vi "CalibrateCurrentDriver.vi"() -> ()   [LabVIEW 2025]
uses:
  <vilib>/Analysis/1siggen.llb/Ramp Pattern by Samples.vi
  <vilib>/Analysis/NI_AALBase.lvlib
  instr.lib/Keithley 648X Series/Keithley 648X Series.lvlib
  <userlib>/_OpenG.lib/time/time.llb/openg_time.lvlib
  <vilib>/Analysis/NI_AALPro.lvlib
panel:
  out "Resistance":dbl format="%#_6p"
  out "intercept":dbl format="%^#_6g"
  out "slope":dbl format="%^#_6g"
  out "XY Graph":cluster{dbl[], "Ramp Pattern":dbl[]}(graph)
  in  "milliseconds to wait":u32
  in  "VISA resource name":refnum<visa-resource-name>
  in  "VSource":refnum<k21>
  in  "nSteps":i32=100 min=2 max=1000 step=1
  in  "MaxVolts":dbl=10.0
  in  "MinVolts":dbl
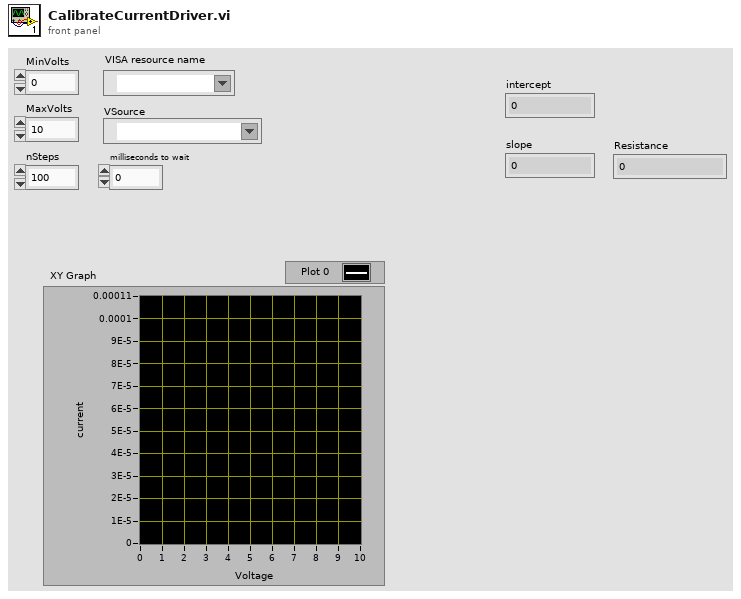
[diagram p1: front panel]
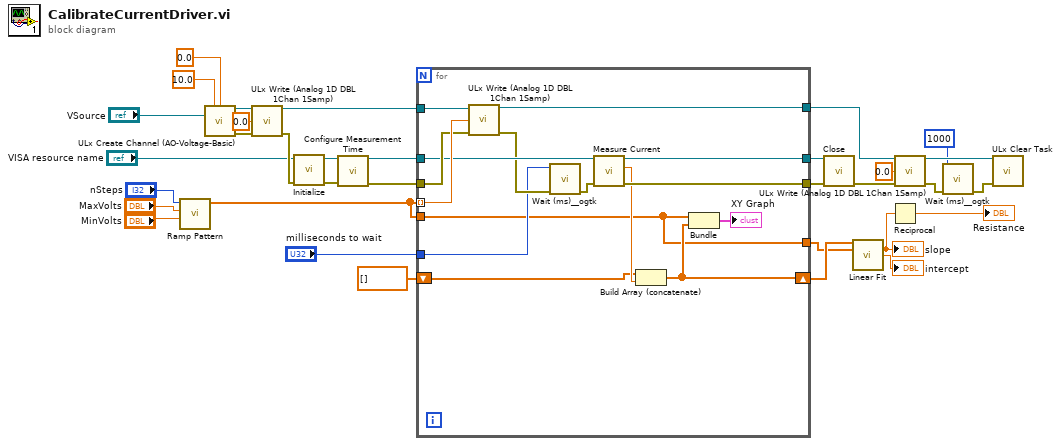
[diagram p0: block diagram]
diagram:
  n1 = call-poly <vilib>:"Ramp Pattern.vi"("start"="MinVolts", "end"="MaxVolts", "samples"="nSteps") -> ("Ramp Pattern"=w13:dbl[])  [unwired: 7 in, 1 out]
  n2 = call <instrlib>:"ULx Create Channel (AO-Voltage-Basic).vi"("maximum value"=10.0, "minimum value"=0.0, "physical channels"="VSource") -> ("task out"=w27:refnum<k24>, "error out"=w26:errorcluster)  [unwired: 11 in]
  n3 = call <instrlib>:"ULx Write (Analog 1D DBL 1Chan 1Samp).vi"("task in"=w27, "data"=0.0, "error in"=w26) -> ("task out"=w18:refnum<k24>, "error out"=w24:errorcluster)  [unwired: 10 in, 1 out]
  n4 = call "Initialize.vi"("error in (no error)"=w24, "VISA resource name"="VISA resource name") -> ("error out"=w21:errorcluster, "VISA resource name out"=w22:refnum<visa-resource-name>)  [unwired: 8 in]
  n5 = call "Configure Measurement Time.vi"("VISA resource name"=w22, "error in (no error)"=w21) -> ("VISA resource name out"=w19:refnum<visa-resource-name>, "error out"=w20:errorcluster)  [unwired: 12 in]
  n6 = for {
    tunnel: w20 -> [w46]
    tunnel: w19 -> [w45]
    tunnel: w18 -> [w48]
    tunnel: w13 -> [w47] mode=indexing
    tunnel: [w43] -> w16
    tunnel: "milliseconds to wait" -> [w41]
    tunnel: [w40] -> w15
    tunnel: [w39] -> w5
    shift-right: [w35] -> w12
    shift-left: dbl[] [] -> [w37]
    tunnel: w13 -> [w34]
    tunnel: [w34] -> w11
    n7 = call <instrlib>:"ULx Write (Analog 1D DBL 1Chan 1Samp).vi"("task in"=w48, "data"=w47, "error in"=w46) -> ("task out"=w39:refnum<k24>, "error out"=w44:errorcluster)  [unwired: 10 in, 1 out]
    n8 = call <userlib>:"Wait (ms)__ogtk.vi"("error in (no error)"=w44, "milliseconds to wait"=w41) -> ("error out"=w42:errorcluster)  [unwired: 8 in, 1 out]
    n9 = call "Measure Current.vi"("VISA resource name"=w45, "error in (no error)"=w42) -> ("VISA resource name out"=w43:refnum<visa-resource-name>, "Measurement"=w38:dbl, "error out"=w40:errorcluster)  [unwired: 11 in]
    n10 = Build Array (concatenate)(w37, w38) -> (w35:dbl[])
    n11 = Bundle("Ramp Pattern"=w34, w35) -> (→"XY Graph":cluster{"Ramp Pattern":dbl[], dbl[]})  [unwired: 1 in]
  }
  n12 = call "Close.vi"("error in (no error)"=w15, "VISA resource name"=w16) -> ("error out"=w4:errorcluster)  [unwired: 9 in]
  n13 = call <vilib>:"Linear Fit.vi"("Y"=w12, "X"=w11) -> ("slope"=w9:dbl, "intercept"=→"intercept":dbl)  [unwired: 9 in, 3 out]
  "slope" <- w9
  n14 = Reciprocal(x=w9) -> (1/x=→"Resistance":dbl)
  n15 = call <instrlib>:"ULx Write (Analog 1D DBL 1Chan 1Samp).vi"("task in"=w5, "data"=0.0, "error in"=w4) -> ("task out"=w6:refnum<k24>, "error out"=w3:errorcluster)  [unwired: 10 in, 1 out]
  n16 = call <userlib>:"Wait (ms)__ogtk.vi"("error in (no error)"=w3, "milliseconds to wait"=u32 1000) -> ("error out"=w2:errorcluster)  [unwired: 8 in, 1 out]
  n17 = call <instrlib>:"ULx Clear Task.vi"("task in"=w6, "error in"=w2) -> ()  [unwired: 13 in, 1 out]
